vi "sc_reset_manipulator.vi"(8 "error in (no error)":errorcluster, 9 "approach? (T = on)":bool, 10 "motion":T1=enum."slow_dualPatch", 11 "visa in":refnum<visa-resource-name>) -> (0 "error out":errorcluster, 3 "visa out":refnum<visa-resource-name>)   [LabVIEW 2015]
uses:
  pipette cleaning/pressure box/cleaning_soft/controls/scientifica_commands.ctl
  controls/scope_motion.ctl
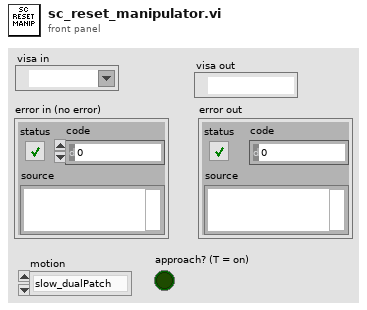
[diagram p1: front panel]
types:
  T1 = typedef "scope_motion.ctl" = enum16{"superSlow", "fast", "slow", "find slice speed", "slow_dualPatch"}
  T2 = typedef "scientifica_commands.ctl" = enum16{"ANGLE", "INSET", "FIRST", "ZERO", "Pz", "P", "absz", "ACC", "TOP", "STOP", "rel", "relz", "abs", "IN", "vj", "APROACH", "OBJS", "OBJU", "OUT", "OBJ", "OBJL", "SET", "OBJD", "STEP", "SETSTEP", "S", "UUX", "UUY", "UUZ"}
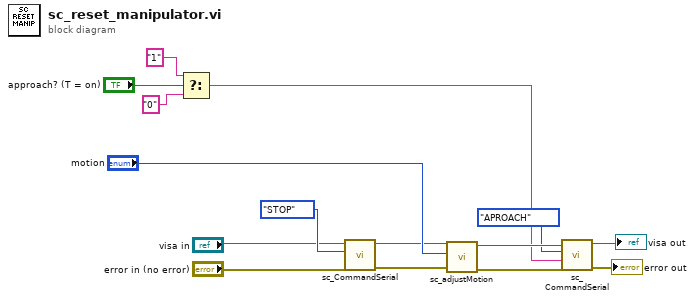
[diagram p0: block diagram]
diagram:
  n1 = Select(t="1" ("argument"), s="approach? (T = on)", f="0" ("argument")) -> (s? t:f=w1:string)
  n2 = call "sc_CommandSerial.vi"("error in (no error)"="error in (no error)", "Scientifica commands"=scientifica_commands."STOP", "VISA handle"="visa in") -> ("error out"=w7:errorcluster, "Dup. VISA handle"=w8:refnum<visa-resource-name>)  [unwired: 5 in, 2 out]
  n3 = call "sc_adjustMotion.vi"("error in (no error)"=w7, "motion"="motion", "VISA handle"=w8) -> ("error out"=w14:errorcluster, "Dup. VISA handle"=w13:refnum<visa-resource-name>)  [unwired: 7 in]
  n4 = call "sc_CommandSerial.vi"("error in (no error)"=w14, "argument"=w1, "Scientifica commands"=scientifica_commands."APROACH", "VISA handle"=w13) -> ("error out"=→"error out":errorcluster, "Dup. VISA handle"=→"visa out":refnum<visa-resource-name>)  [unwired: 4 in, 2 out]
